vi "Potting Data - Address Pads.vi"(10 "Address Pads Selection":cluster{"Top":bool, "Bottom":bool}, 11 "Address Pads Data":T2) -> (3 "Potting Lines":T1[](array[typedef]))   [LabVIEW 2011]
uses:
  Shared Components/Utils/Type Definitions/Multi-Fiducial Image.ctl
  Shared Components/Vec3d Class/Vec3d Class.lvclass
  Shared Components/Utils/Type Definitions/Physical Image.ctl
  <vilib>/vision/Image Controls.llb/IMAQ Image.ctl
  Shared Components/Utils/Type Definitions/Fiducial with Source.ctl
  Shared Components/Utils/Type Definitions/3d Line.ctl
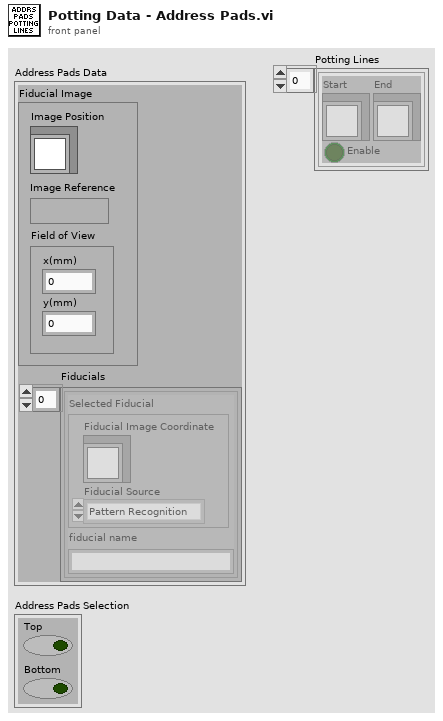
[diagram p1: front panel]
types:
  T1 = typedef "3d Line.ctl" = cluster{"Start":refnum<class "Vec3d Class.lvclass">, "End":refnum<class "Vec3d Class.lvclass">, "Enable":bool}
  T2 = typedef "Multi-Fiducial Image.ctl" = cluster{"Fiducial Image":T3, "Fiducials":cluster{"Selected Fiducial":T5, "fiducial name":string}[]}
  T3 = typedef "Physical Image.ctl" = cluster{"Image Position":refnum<class "Vec3d Class.lvclass">, "Image Reference":T4, "Field of View":cluster{"x(mm)":dbl, "y(mm)":dbl}}
  T4 = typedef "IMAQ Image.ctl" = refnum<image>
  T5 = typedef "Fiducial with Source.ctl" = cluster{"Fiducial Image Coordinate":refnum<class "Vec3d Class.lvclass">, "Fiducial Source":enum16{"Pattern Recognition", "User", "Error", "Default"}}
  T6 = cluster{"Selected Fiducial":T5, "fiducial name":string}[]
  T7 = cluster{"Selected Fiducial":T5, "fiducial name":string}
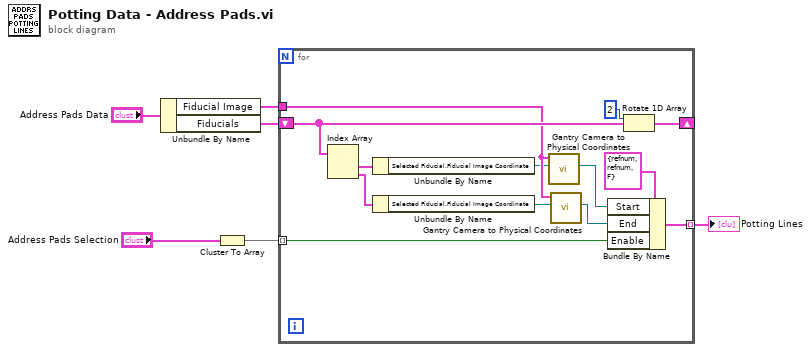
[diagram p0: block diagram]
diagram:
  n1 = Unbundle By Name("Address Pads Data") -> ("Fiducial Image"=w2:T3, "Fiducials"=w4:T6)
  n2 = Cluster To Array(cluster="Address Pads Selection") -> (array=w5:bool[])
  n3 = for {
    tunnel: w5 -> [w7] mode=indexing
    shift-right: [w17] -> _
    shift-left: w4 -> [w18]
    tunnel: w2 -> [w16]
    tunnel: [w8] -> w1 mode=indexing
    n4 = Index Array(array=w18) -> (element #1=w14:T7, element #2=w15:T7)  [unwired: 2 in]
    n5 = Unbundle By Name(w14) -> ("Selected Fiducial.Fiducial Image Coordinate"=w12:refnum<class "Vec3d Class.lvclass">)
    n6 = Unbundle By Name(w15) -> ("Selected Fiducial.Fiducial Image Coordinate"=w10:refnum<class "Vec3d Class.lvclass">)
    n7 = call "Gantry Camera to Physical Coordinates.vi"("Image Coordinate"=w12, "Physical Image"=w16) -> ("Global Coordinate"=w11:refnum<class "Vec3d Class.lvclass">)  [unwired: 7 in, 2 out]
    n8 = call "Gantry Camera to Physical Coordinates.vi"("Image Coordinate"=w10, "Physical Image"=w16) -> ("Global Coordinate"=w9:refnum<class "Vec3d Class.lvclass">)  [unwired: 7 in, 2 out]
    n9 = Bundle By Name(cluster=T1 {"Start"=refnum, "End"=refnum, "Enable"=FALSE} ("3D Line"), "Start"=w11, "End"=w9, "Enable"=w7) -> (w8:T1)
    n10 = Rotate 1D Array(1:w18, 2:2 ("n")) -> (0:w17:T6)
  }
  "Potting Lines" <- w1
